vi "tStat2021_eng.vi"() -> ()   [LabVIEW 2016]
doc: "This VI was designed to demonstrate typical usage of sub VIs containing the more common 335 functions. The VI Initializes the instrument, allows the user to determine if heater output control parameters and setpoint values are sent, takes a single sensor reading, and then closes the instrument."
uses:
  <instrlib>/Lake Shore 335/Public/Data/Sensor Data (Single Reading).vi
  <instrlib>/Lake Shore 335/Lake Shore 335.lvlib
panel:
  out "Plot is saved":bool
  in  "string":string="Введите название образца"
  in  "file path (use dialog)":path=path "C:/Users/User_Lab2/Desktop/Lakeshore/Temp_Temperature"
  out "String":string
  out "Boolean":bool
  in  "Stop":bool
  out "Current sample temperature, K":dbl format="%.4f"
  out "Сurrent power value, %":dbl caption="Power" format="%.1f"
  out "Temperature on cryohead, K":dbl format="%.4f"
  out "Protocol of temperature changes since start":cluster{"Y":dbl[], "Y":dbl[]}[](graph) caption="Протокол изменения температуры \nс момента запуска программы"
  in  "Heater power control":T1(radio)
  in  "Build Graph":bool
  out "Temperature (T)":dbl(graph)
  in  "Set":bool
  in  "Set sample temperature, K":dbl format="%.4f"
  # "Power value is indicated for a given range\nLOW = 0.1 * MEDIUM = 0.01 * HIGH"
  # "Plot of current temperature"
  # "FSRC"
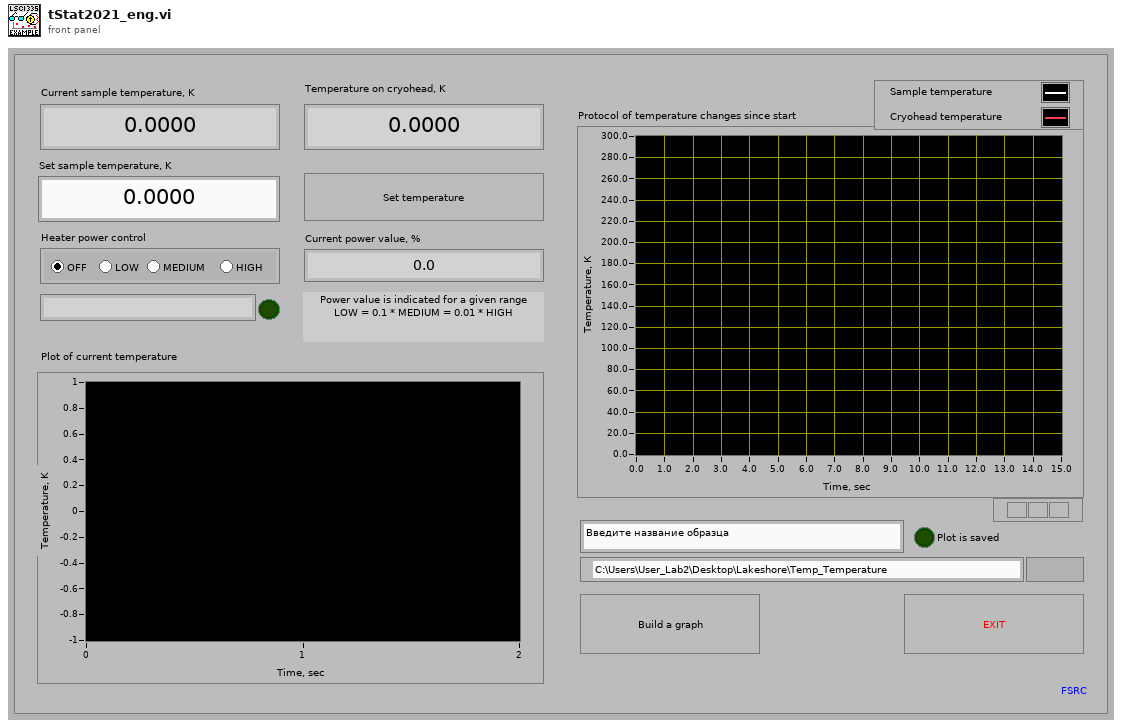
[diagram p1: front panel]
types:
  T1 = enum32{"Radio Selection 1", "Radio Selection 2", "Radio Selection 3", "Radio Selection 4"}
  T2 = cluster{"Baud Rate":u32, "Parity":u16, "Data Bits":u16, "Stop Bits":u16, "Flow Control":u16}
  T3 = enum16{"open", "replace", "create", "open or create", "replace or create", "replace or create with confirmation"}
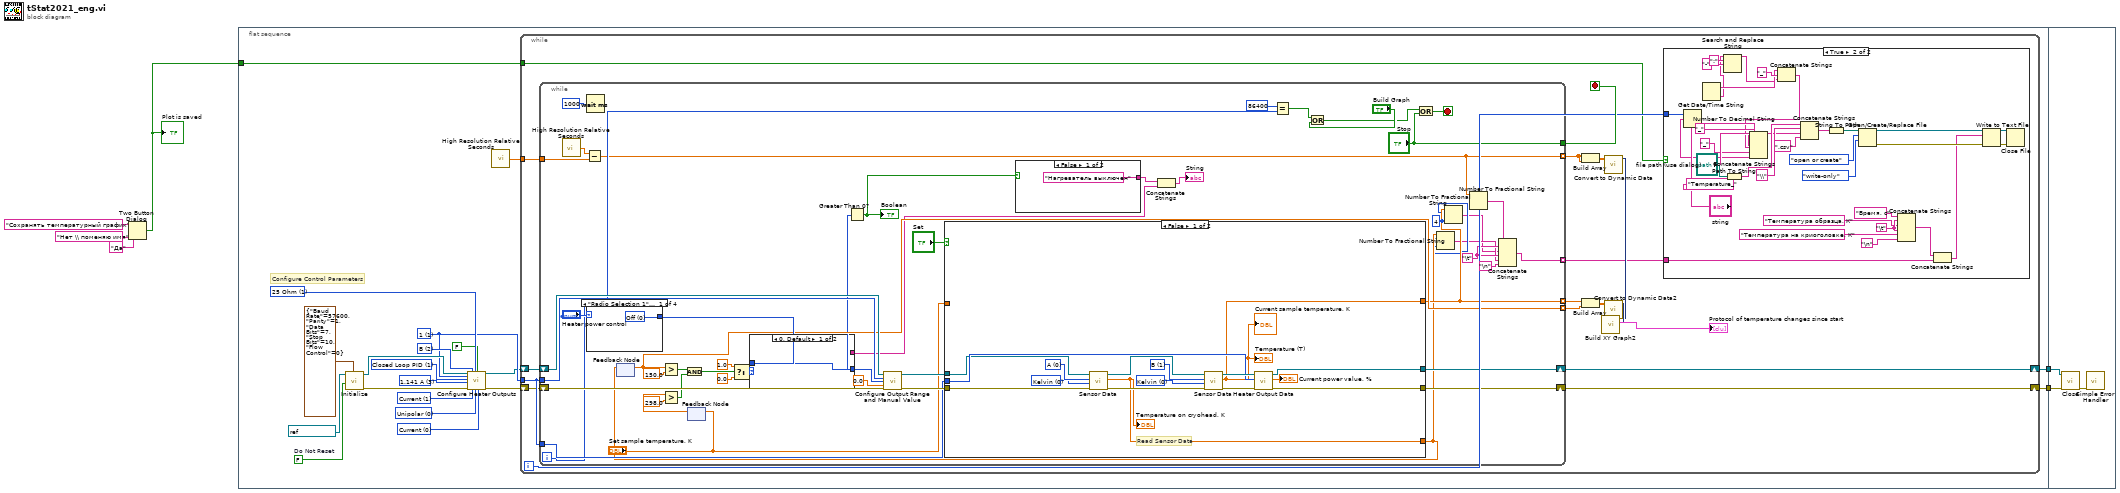
[diagram p0: block diagram]
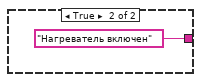
[diagram p3: hidden frame]
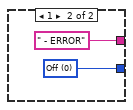
[diagram p4: hidden frame]
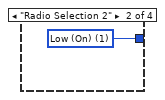
[diagram p5: hidden frame]
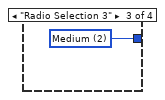
[diagram p6: hidden frame]
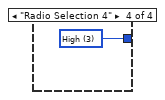
[diagram p7: hidden frame]
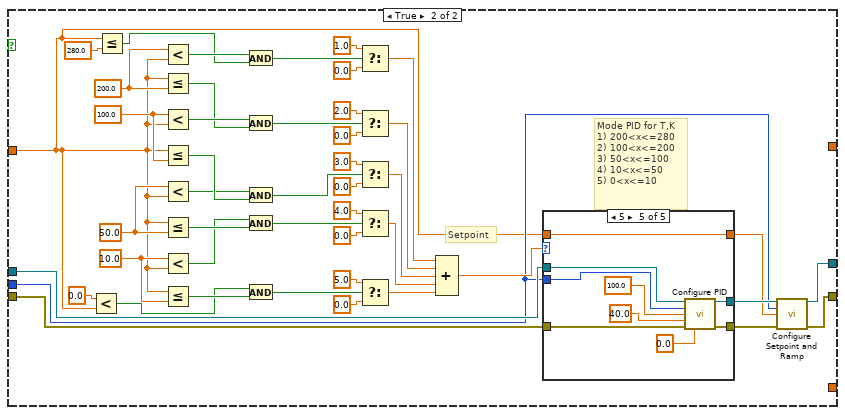
[diagram p8: hidden frame]
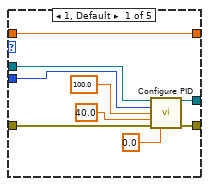
[diagram p9: hidden frame]
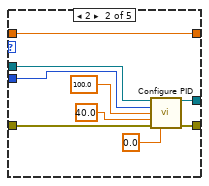
[diagram p10: hidden frame]
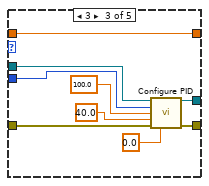
[diagram p11: hidden frame]
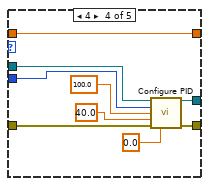
[diagram p12: hidden frame]
diagram:
  n1 = Two Button Dialog(message="Сохранять температурный график?", 1:"Нет \\ поменяю имя" ("F button name (\"Cancel\")"), 2:"Да" ("T button name (\"OK\")")) -> (T button?=w3:bool)
  "Plot is saved" <- w3
  n2 = flat-sequence {
    tunnel: [w23] -> w2
    tunnel: [w22] -> w1
    tunnel: w3 -> [w7]
    tunnel: w2 -> [w244]
    tunnel: w1 -> [w243]
    frame #0 {
      w15 = u16 1 items=["25 Ohm"=1, "50 Ohm"=2] ("Heater Resistance (1:25 Ohm)")
      w16 = u16 2 items=["None", "A", "B"] ("Input (0:None)")
      w11 = u16 1 items=["1"=1, "2"=2] ("Heater Output (1:1)")
      w17 = u16 1 items=["Off", "Closed Loop PID", "Zone", "Open Loop", "Monitor Out", "Warmup Supply"] ("Mode (0:Off)")
      w18 = u16 3 items=["User Specified", "0.707 A", "1.0 A", "1.141 A", "1.732 A"] ("Max Current (0:User Specified)")
      w21 = u16 0 items=["Current", "Voltage"] ("Output Type (0:Current)")
      w20 = u16 0 items=["Unipolar", "Bipolar"] ("Polarity (0:Unipolar)")
      w19 = u16 1 items=["Current"=1, "Power"=2] ("Heater Out Display (1:Current)")
      w25 = FALSE  # Do Not Reset
      # "Configure Control Parameters"
      n3 = call <instrlib>:"Initialize.vi"("Serial Configuration"=T2 {"Baud Rate"=57600, "Parity"=1, "Data Bits"=7, "Stop Bits"=10, "Flow Control"=0}, "Reset (True)"=w25, "VISA resource name"=refnum<visa-resource-name> "Lakeshore") -> ("error out"=w12:errorcluster, "VISA resource name out"=w13:refnum<visa-resource-name>)  [unwired: 7 in]
      n4 = call <instrlib>:"Configure Heater Outputs.vi"("VISA resource name"=w13, "Heater Output (1:1)"=w11, "Mode (0:Off)"=w17, "Max Current (0:User Specified)"=w18, "error in (no error)"=w12, "Input (0:None)"=w16, "Heater Out Display (1:Current)"=w19, "Heater Resistance (1:25 Ohm)"=w15, "Polarity (0:Unipolar)"=w20, "Power Up Enable (F: Off)"=FALSE, "Output Type (0:Current)"=w21) -> ("VISA resource name out"=w9:refnum<visa-resource-name>, "error out"=w10:errorcluster)  [unwired: 7 in]
      n5 = call <vilib>:"High Resolution Relative Seconds.vi"() -> ("relative seconds"=w8:dbl)
      n6 = while {
        tunnel: w11 -> [w42]
        shift-right: [w43] -> w22
        shift-left: w10 -> [w41]
        shift-right: [w44] -> w23
        shift-left: w9 -> [w40]
        tunnel: w8 -> [w38]
        tunnel: w7 -> [w27]
        i -> [w29]
        stop <- w39 stop-if-true
        n7 = while {
          shift-right: [w125] -> w44
          shift-left: w40 -> [w123]
          shift-right: [w126] -> w43
          shift-left: w41 -> [w122]
          tunnel: w42 -> [w119]
          tunnel: w42 -> [w117]
          tunnel: [w85] -> w33 mode=indexing
          tunnel: w38 -> [w114]
          tunnel: [w86] -> w37 mode=indexing
          tunnel: ["Stop"] -> w39
          tunnel: [w102] -> w32 mode=indexing
          tunnel: [w79] -> w28 mode=indexing
          i -> [w93]
          stop <- w113 stop-if-true
          w83 = i16 4 ("precision (6)")
          w88 = "\t" ("Tab")
          n8 = call <vilib>:"High Resolution Relative Seconds.vi"() -> ("relative seconds"=w115:dbl)
          n9 = Subtract(x=w115, y=w114) -> (x-y=w86:dbl)
          n10 = Wait (ms)(milliseconds to wait=u32 1000) -> ()  [unwired: 1 out]
          n11 = case shown="\"Radio Selection 1\", Default" "Heater power control" {
            tunnel: [w132 w133 w134 w135] -> w103
            frame "Radio Selection 1", Default {
              w132 = u16 0 items=["Off", "Low (On)", "Medium", "High"] ("Range (0:Off)")
            }
            frame "Radio Selection 2" {
              w133 = u16 1 items=["Off", "Low (On)", "Medium", "High"] ("Range (0:Off)")
            }
            frame "Radio Selection 3" {
              w134 = u16 2 items=["Off", "Low (On)", "Medium", "High"] ("Range (0:Off)")
            }
            frame "Radio Selection 4" {
              w135 = u16 3 items=["Off", "Low (On)", "Medium", "High"] ("Range (0:Off)")
            }
          }
          n12 = feedback #1() -> (w102:dbl)  [unwired: 1 in]
          n13 = Greater?(x=w102, y=150.0) -> (0:w108:bool)
          n14 = feedback-in #2("Set sample temperature, K") -> ()
          n15 = feedback #2() -> (w101:dbl)  [unwired: 1 in]
          n16 = Greater?(x=w101, y=298.0) -> (0:w105:bool)
          n17 = And(x=w108, y=w105) -> (x .and. y?=w109:bool)
          n18 = Select(t=1.0, s=w109, f=0.0) -> (s? t:f=w107:dbl)
          n19 = case shown="0, Default" w107 {
            tunnel: [w129 w131] -> w99
            tunnel: w103 -> [w129 _]
            tunnel: [_ " - ERROR" ("String")] -> w95
            frame 0, Default {
            }
            frame 1 {
              w131 = u16 0 items=["Off", "Low (On)", "Medium", "High"] ("Range (0:Off)")
            }
          }
          n20 = Greater Than 0?(x=w99) -> (x > 0?=w97:bool)
          "Boolean" <- w97
          n21 = call <instrlib>:"Configure Output Range and Manual Value.vi"("VISA resource name"=w123, "Heater Output (1:1)"=w119, "Range (0:Off)"=w99, "Manual Output (0.00 %)"=0.0, "error in (no error)"=w122) -> ("VISA resource name out"=w121:refnum<visa-resource-name>, "error out"=w120:errorcluster)  [unwired: 9 in]
          n22 = case shown="False" "Set" {
            tunnel: w121 -> [w142 w159]
            tunnel: w120 -> [w141 w160]
            tunnel: [w151 w156] -> w125
            tunnel: [w150 w155] -> w126
            tunnel: w117 -> [w146 w154]
            tunnel: [w144 _] -> w85
            tunnel: [w136 _] -> w84
            tunnel: "Set sample temperature, K" -> [_ w152]
            frame False {
              w137 = u16 0 items=["Kelvin", "Celsius", "Sensor Units"] ("Data Source (0:Kelvin)")
              w138 = u16 0 items=["A", "B"] ("Input (0:A)")
              w145 = u16 1 items=["A", "B"] ("Input (0:A)")
              w149 = u16 0 items=["Kelvin", "Celsius", "Sensor Units"] ("Data Source (0:Kelvin)")
              # "Read Sensor Data"
              n23 = call-poly <instrlib>:"Sensor Data.vi"("error in (no error)"=w141, "Data Source (0:Kelvin)"=w137, "Input (0:A)"=w138, "VISA resource name"=w142) -> ("error out"=w140:errorcluster, "Sensor Data"=w136:dbl, "VISA resource name out"=w139:refnum<visa-resource-name>)  [unwired: 5 in]
              "Temperature on cryohead, K" <- w136
              n24 = call-poly <instrlib>:"Sensor Data.vi"("error in (no error)"=w140, "Data Source (0:Kelvin)"=w149, "Input (0:A)"=w145, "VISA resource name"=w139) -> ("error out"=w147:errorcluster, "Sensor Data"=w144:dbl, "VISA resource name out"=w148:refnum<visa-resource-name>)  [unwired: 5 in]
              "Temperature (T)" <- w144
              "Current sample temperature, K" <- w144
              n25 = call <instrlib>:"Heater Output Data.vi"("error in (no error)"=w147, "Heater Output (1:1)"=w146, "VISA resource name"=w148) -> ("error out"=w150:errorcluster, "Output Value"=→"Сurrent power value, %":dbl, "VISA resource name out"=w151:refnum<visa-resource-name>)  [unwired: 6 in]
            }
            frame True {
              w162 = 10.0 ("x")
              w163 = 50.0 ("x")
              w164 = 100.0 ("x")
              w165 = 200.0 ("x")
              # "Mode PID for T,K\n1) 200<x<=280\n2) 100<x<=200\n3) 50<x<=100\n4) 10<x<=50\n5) 0<x<=10"
              # "Setpoint"
              n26 = Less?(x=0.0, y=w152) -> (x < y?=w171:bool)
              n27 = Less Or Equal?(x=w152, y=280.0 ("x")) -> (x <= y?=w167:bool)
              n28 = Less?(x=w165, y=w152) -> (x < y?=w168:bool)
              n29 = Less Or Equal?(x=w152, y=w165) -> (x <= y?=w169:bool)
              n30 = Less?(x=w164, y=w152) -> (x < y?=w170:bool)
              n31 = Less Or Equal?(x=w152, y=w164) -> (x <= y?=w176:bool)
              n32 = Less?(x=w163, y=w152) -> (x < y?=w175:bool)
              n33 = Less Or Equal?(x=w152, y=w163) -> (x <= y?=w174:bool)
              n34 = Less?(x=w162, y=w152) -> (x < y?=w173:bool)
              n35 = Less Or Equal?(x=w152, y=w162) -> (x <= y?=w172:bool)
              n36 = And(x=w168, y=w167) -> (x .and. y?=w184:bool)
              n37 = And(x=w170, y=w169) -> (x .and. y?=w178:bool)
              n38 = And(x=w175, y=w176) -> (x .and. y?=w179:bool)
              n39 = And(x=w173, y=w174) -> (x .and. y?=w181:bool)
              n40 = And(x=w171, y=w172) -> (x .and. y?=w180:bool)
              n41 = Select(t=1.0, s=w184, f=0.0) -> (s? t:f=w189:dbl)
              n42 = Select(t=2.0, s=w178, f=0.0) -> (s? t:f=w188:dbl)
              n43 = Select(t=3.0, s=w179, f=0.0) -> (s? t:f=w187:dbl)
              n44 = Select(t=4.0, s=w181, f=0.0) -> (s? t:f=w186:dbl)
              n45 = Select(t=5.0, s=w180, f=0.0) -> (s? t:f=w177:dbl)
              n46 = Compound Arithmetic op=ADD(w189, w188, w187, w186, w177) -> (w185:dbl)
              n47 = case shown="5" w185 {
                tunnel: w154 -> [w206 w215 w224 w233 w242]
                tunnel: w159 -> [w202 w209 w220 w229 w235]
                tunnel: w160 -> [w201 w208 w219 w228 w238]
                tunnel: [w200 w211 w218 w227 w237] -> w158
                tunnel: [w199 w210 w217 w226 w236] -> w157
                tunnel: w152 -> [w198 w207 w216 w225 w234]
                tunnel: [w198 w207 w216 w225 w234] -> w153
                frame 1, Default {
                  n48 = call <instrlib>:"Configure PID.vi"("VISA resource name"=w202, "Output's Control Loop (1:1)"=w206, "Gain (P) (50.0)"=100.0, "Reset (I) (20.0)"=40.0, "error in (no error)"=w201, "Rate (D) (0.0 %)"=0.0) -> ("VISA resource name out"=w200:refnum<visa-resource-name>, "error out"=w199:errorcluster)  [unwired: 8 in]
                }
                frame 2 {
                  n49 = call <instrlib>:"Configure PID.vi"("VISA resource name"=w209, "Output's Control Loop (1:1)"=w215, "Gain (P) (50.0)"=100.0, "Reset (I) (20.0)"=40.0, "error in (no error)"=w208, "Rate (D) (0.0 %)"=0.0) -> ("VISA resource name out"=w211:refnum<visa-resource-name>, "error out"=w210:errorcluster)  [unwired: 8 in]
                }
                frame 3 {
                  n50 = call <instrlib>:"Configure PID.vi"("VISA resource name"=w220, "Output's Control Loop (1:1)"=w224, "Gain (P) (50.0)"=100.0, "Reset (I) (20.0)"=40.0, "error in (no error)"=w219, "Rate (D) (0.0 %)"=0.0) -> ("VISA resource name out"=w218:refnum<visa-resource-name>, "error out"=w217:errorcluster)  [unwired: 8 in]
                }
                frame 4 {
                  n51 = call <instrlib>:"Configure PID.vi"("VISA resource name"=w229, "Output's Control Loop (1:1)"=w233, "Gain (P) (50.0)"=100.0, "Reset (I) (20.0)"=40.0, "error in (no error)"=w228, "Rate (D) (0.0 %)"=0.0) -> ("VISA resource name out"=w227:refnum<visa-resource-name>, "error out"=w226:errorcluster)  [unwired: 8 in]
                }
                frame 5 {
                  n52 = call <instrlib>:"Configure PID.vi"("VISA resource name"=w235, "Output's Control Loop (1:1)"=w242, "Gain (P) (50.0)"=100.0, "Reset (I) (20.0)"=40.0, "error in (no error)"=w238, "Rate (D) (0.0 %)"=0.0) -> ("VISA resource name out"=w237:refnum<visa-resource-name>, "error out"=w236:errorcluster)  [unwired: 8 in]
                }
              }
              n53 = call <instrlib>:"Configure Setpoint and Ramp.vi"("VISA resource name"=w158, "Output's Control Loop (1:1)"=w154, "Setpoint (0.0000)"=w153, "error in (no error)"=w157) -> ("VISA resource name out"=w156:refnum<visa-resource-name>, "error out"=w155:errorcluster)  [unwired: 10 in]
            }
          }
          n54 = feedback-in #1(w84) -> ()
          n55 = case shown="False" w97 {
            tunnel: ["Нагреватель выключен" ("String") "Нагреватель включен" ("String")] -> w96
            frame False {
            }
            frame True {
            }
          }
          n56 = Concatenate Strings(w96, w95) -> (→"String":string)
          n57 = Equal?(x=86400, y=w93) -> (x = y?=w91:bool)
          n58 = Or(x=w91, y="Build Graph") -> (x .or. y?=w89:bool)
          n59 = Or(x=w89, y="Stop") -> (x .or. y?=w113:bool)
          n60 = Number To Fractional String(number=w84, precision (6)=w83) -> (F-format string=w82:string)  [unwired: 2 in]
          n61 = Number To Fractional String(number=w85, precision (6)=w83) -> (F-format string=w81:string)  [unwired: 2 in]
          n62 = Number To Fractional String(number=w86) -> (F-format string=w80:string)  [unwired: 3 in]
          n63 = Concatenate Strings(w80, w88, w81, w88, w82, "\n") -> (w79:string)
        }
        n64 = Build Array(w37, w37) -> (w36:dbl[][])
        n65 = Build Array(w33, w32) -> (w35:dbl[][])
        n66 = call "Convert to Dynamic Data"("2D Array"=w36) -> ("Dynamic Data Type"=w30:dynamicdata)  [unwired: 3 in]
        n67 = call "Convert to Dynamic Data2"("2D Array"=w35) -> ("Dynamic Data Type"=w31:dynamicdata)  [unwired: 3 in]
        n68 = call "Build XY Graph2"("Y Input"=w31, "X Input"=w30) -> ("XY Graph"=→"Protocol of temperature changes since start":cluster{"X":dbl[], "Y":dbl[]}[])  [unwired: 8 in, 1 out]
        n69 = case shown="True" w27 {
          tunnel: w29 -> [_ w66]
          tunnel: w28 -> [_ w61]
          frame False {
          }
          frame True {
            w65 = "\t" ("Tab")
            n70 = Number To Decimal String(number=w66) -> (decimal integer string=w50:string)  [unwired: 1 in]
            n71 = Get Date/Time String() -> (date string=w52:string, time string=w46:string)  [unwired: 3 in]
            n72 = Search and Replace String(input string=w46, search string=":", replace string="-" ("replace string (\"\")")) -> (result string=w45:string)  [unwired: 5 in, 3 out]
            n73 = Path To String(path="file path (use dialog)") -> (string=w71:string)
            n74 = Concatenate Strings(w52, "_" ("string"), w45) -> (w51:string)
            n75 = Concatenate Strings("Temperature_" ("string"), "string", "_" ("string"), w51, "_" ("string"), w50) -> (w56:string)
            n76 = Concatenate Strings(w71, "\\" ("string"), w56, ".csv" ("string")) -> (w70:string)
            n77 = String To Path(string=w70) -> (path=w69:path)
            n78 = Open/Create/Replace File(file path (use dialog)=w69, operation (0:open)=T3."open or create", access (0:read/write)=enum16{"read/write", "read-only", "write-only"}."write-only") -> (refnum out=w76:refnum<file>, error out=w75:errorcluster)  [unwired: 3 in, 1 out]
            n79 = Concatenate Strings("Время, с" ("string"), w65, "Температура образца, К" ("string"), w65, "Температура на криоголовке, К" ("string"), "\n") -> (w59:string)
            n80 = Concatenate Strings(w59, w61) -> (w58:string)
            n81 = Write to Text File(file (use dialog)=w76, text=w58, error in=w75) -> (refnum out=w73:refnum<file>, error out=w74:errorcluster)  [unwired: 1 in, 1 out]
            n82 = Close File(refnum=w73, error in=w74) -> ()  [unwired: 2 out]
          }
        }
      }
    }
    frame #1 {
      n83 = call <instrlib>:"Close.vi"("error in (no error)"=w243, "VISA resource name"=w244) -> ("error out"=w245:errorcluster)  [unwired: 9 in]
      n84 = call <vilib>:"Simple Error Handler.vi"("error in (no error)"=w245) -> ()  [unwired: 4 in, 5 out]
    }
  }
